vi "degrees-to-radians.vi"() -> ()   [LabVIEW 2025]
panel:
  out "radians":dbl
  in  "180":dbl
  in  "degree":dbl
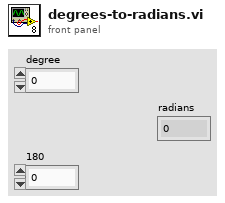
[diagram p1: front panel]
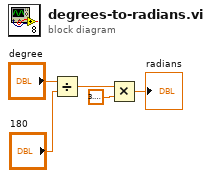
[diagram p0: block diagram]
diagram:
  n1 = Divide(x="degree", y="180") -> (x/y=w3:dbl)
  n2 = Multiply(x=w3, y=3.141592653589793) -> (x*y=→"radians":dbl)
